vi "FTW-Connector-QueryActorInstanceStatus.vi"(0 "FTW Actor Connector Type":refnum<class "FTW-Actor-Connector.lvclass">, 5 "Timeout":i32=100 format="%dmsec", 11 "error in":errorcluster) -> (4 "FTW Actor Connector":refnum<class "FTW-Actor-Connector.lvclass">, 6 "Roundtrip Time":dbl format="%.6fsec", 15 "error out":errorcluster)   [LabVIEW 2014, in "FTW-Actor-Connector.lvclass"]
doc: "Performs a \"cold call\" to connect to a running Actor Instance at the given Instance Inbox Address. Normally, this method is wrapped by a \"Construct\" method in each specific Actor Connector subclass."
uses:
  FTW-Actor-Connector.lvclass
panel:
  # "Inputs"
  # "Outputs"
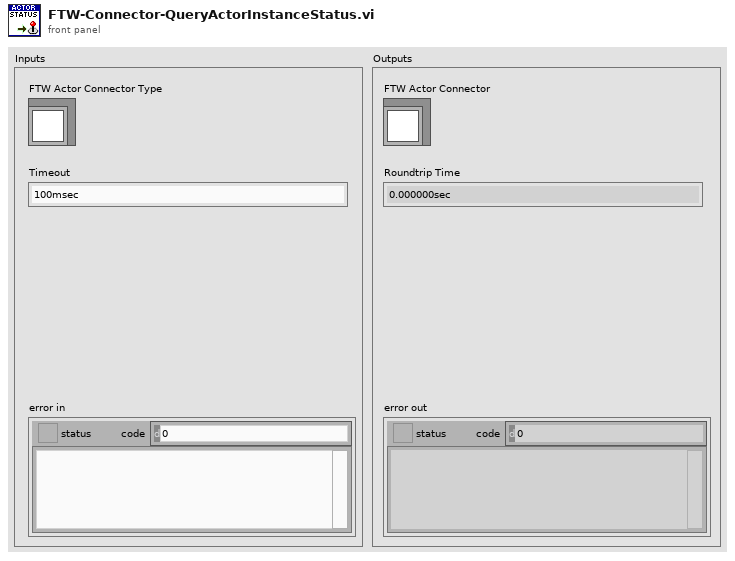
[diagram p1: front panel]
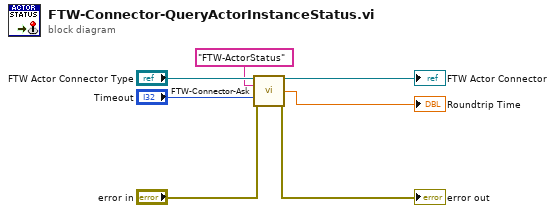
[diagram p0: block diagram]
diagram:
  n1 = call "FTW-Connector-Ask.vi"("FTW Actor Connector"="FTW Actor Connector Type", "Request Header"="FTW-ActorStatus", "Timeout"="Timeout", "error in"="error in") -> ("FTW Actor Connector out"=→"FTW Actor Connector":refnum<class "FTW-Actor-Connector.lvclass">, "Roundtrip Time"=→"Roundtrip Time":dbl, "error out"=→"error out":errorcluster)  [unwired: 8 in, 1 out]
